vi "NetworkStreamProcess.vi"(0 "WaveformConfiguration":T1, 11 "error in (no error)":errorcluster) -> ()   [LabVIEW 2017]
uses:
  <vilib>/NI/DCAF/Modules/FPGAWaveform/execution/Export.ctl
  StreamState.ctl
  StreamHeader.ctl
  globals.vi
  <vilib>/NI/DCAF/Modules/FPGAWaveform/execution/WaveformAcq runtime.lvclass
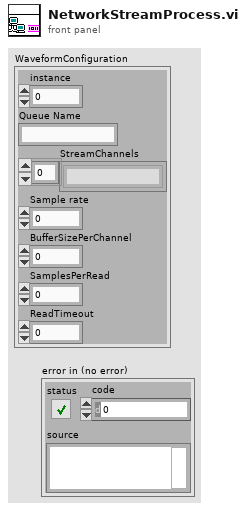
[diagram p1: front panel]
types:
  T1 = typedef "WaveformAcq runtime.lvclass/Export.ctl" = cluster{"instance":i32, "Queue Name":string, "StreamChannels":string[], "Sample rate":i32, "BufferSizePerChannel":i32, "SamplesPerRead":i32, "ReadTimeout":dbl}
  T2 = typedef "StreamHeader.ctl" = cluster{"Channels":string[], "SampleRate":i32}
  T3 = typedef "StreamState.ctl" = enum16{"Idle", "Listening", "Header", "Streaming", "Disconnecting"}
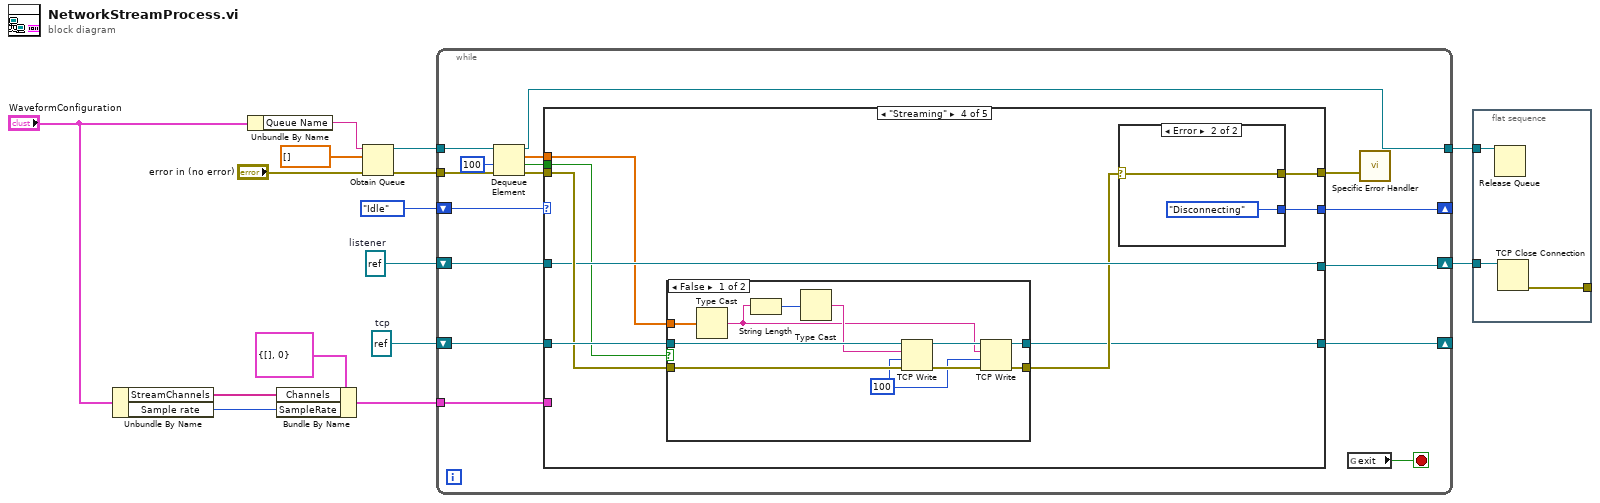
[diagram p0: block diagram]
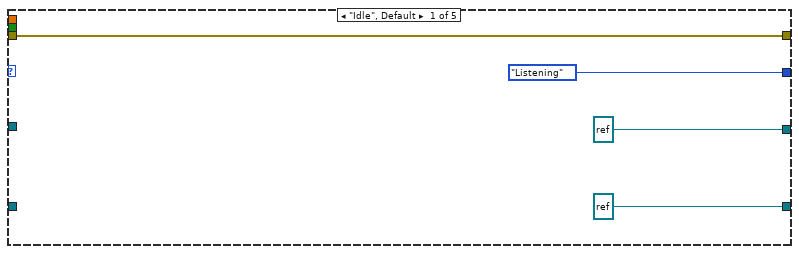
[diagram p2: hidden frame]
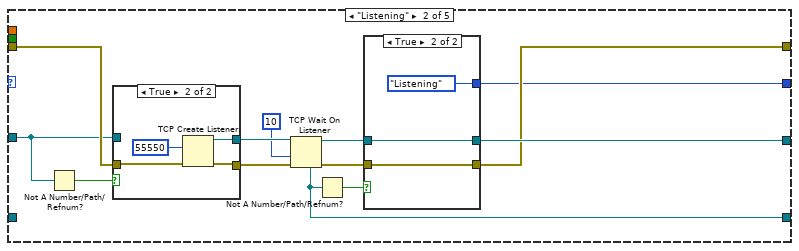
[diagram p3: hidden frame]
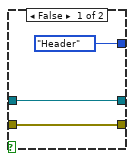
[diagram p4: hidden frame]
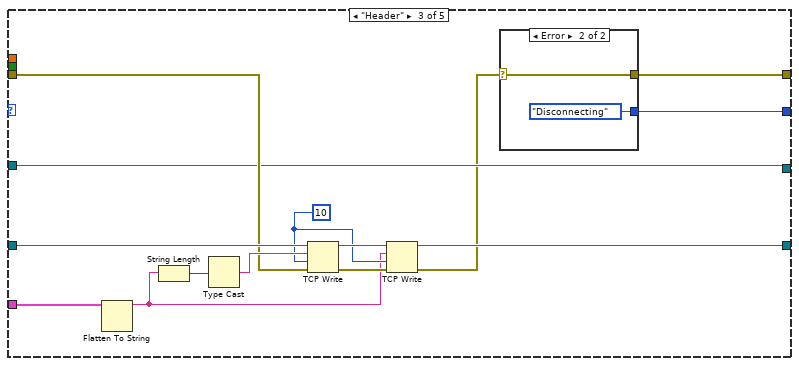
[diagram p6: hidden frame]
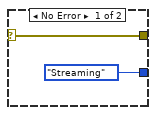
[diagram p7: hidden frame]
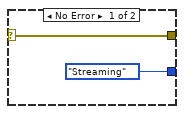
[diagram p8: hidden frame]
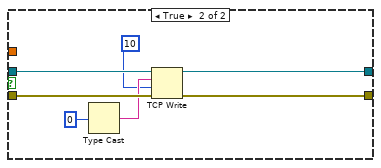
[diagram p9: hidden frame]
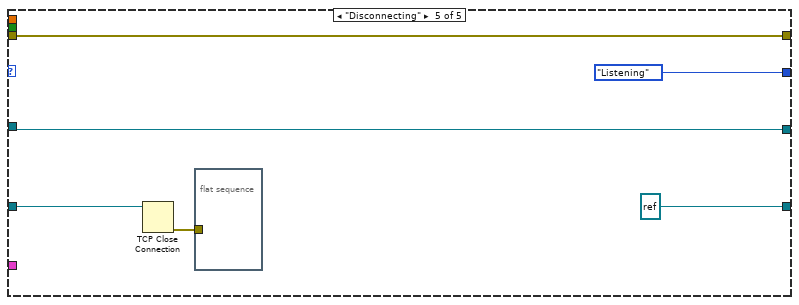
[diagram p10: hidden frame]
diagram:
  w8 = refnum<k5> refnum  # tcp
  w9 = refnum<k5> refnum  # listener
  n1 = Unbundle By Name("WaveformConfiguration") -> ("StreamChannels"=w3:string[], "Sample rate"=w2:i32)
  n2 = Unbundle By Name("WaveformConfiguration") -> ("Queue Name"=w7:string)
  n3 = Bundle By Name(cluster=T2 {"Channels"=[], "SampleRate"=0} ("StreamHeader"), "Channels"=w3, "SampleRate"=w2) -> (w4:T2)
  n4 = Obtain Queue(name (unnamed)=w7, element data type=sgl[] [], error in (no error)="error in (no error)") -> (queue out=w13:refnum<queue>, error out=w14:errorcluster)  [unwired: 2 in, 1 out]
  n5 = while {
    tunnel: w13 -> [w31]
    tunnel: w14 -> [w30]
    tunnel: [w28] -> w15
    shift-right: [w24] -> _
    shift-left: StreamState."Idle" ("StreamState") -> [w26]
    shift-right: [w19] -> w1
    shift-left: w9 -> [w22]
    shift-right: [w18] -> _
    shift-left: w8 -> [w17]
    tunnel: w4 -> [w16]
    stop <- w27 stop-if-true
    n6 = Dequeue Element(queue=w31, timeout in ms (-1)=100, error in (no error)=w30) -> (queue out=w28:refnum<queue>, element=w20:sgl[], timed out?=w21:bool, error out=w25:errorcluster)
    n7 = case shown="\"Streaming\"" w26 {
      tunnel: w25 -> [w32 w47 w71 w86 w111]
      tunnel: [StreamState."Listening" ("StreamState") w36 w67 w85 StreamState."Listening" ("StreamState")] -> w24
      tunnel: [w32 w37 w63 w80 w111] -> w23
      tunnel: w22 -> [_ w46 w65 w84 w110]
      tunnel: w21 -> [_ _ _ w83 _]
      tunnel: w20 -> [_ _ _ w82 _]
      tunnel: [refnum<k5> refnum ("listener ID") w39 w65 w84 w110] -> w19
      tunnel: [refnum<k5> refnum ("listener ID") w38 w66 w79 refnum<k5> refnum ("tcp")] -> w18
      tunnel: w17 -> [_ _ w74 w87 w115]
      tunnel: w16 -> [_ _ w62 _ _]
      frame "Idle", Default {
      }
      frame "Listening" {
        n8 = Not A Number/Path/Refnum?(number/path/refnum=w46) -> (NaN/Path/Refnum?=w48:bool)
        n9 = case shown="True" w48 {
          tunnel: w47 -> [w55 w60]
          tunnel: [w56 w59] -> w45
          tunnel: w46 -> [w56 _]
          tunnel: [w55 w58] -> w44
          frame False {
          }
          frame True {
            n10 = TCP Create Listener(8:w60, 10:u16 55550 ("port")) -> (0:w58:errorcluster, 3:w59:refnum<k5>)  [unwired: 3 in, 1 out]
          }
        }
        n11 = TCP Wait On Listener(8:w44, 9:10 ("timeout ms (wait forever: -1)"), 11:w45) -> (0:w41:errorcluster, 3:w40:refnum<k5>, 4:w38:refnum<k5>)  [unwired: 1 in, 2 out]
        n12 = Not A Number/Path/Refnum?(number/path/refnum=w38) -> (NaN/Path/Refnum?=w42:bool)
        n13 = case shown="True" w42 {
          tunnel: w41 -> [w49 w53]
          tunnel: w40 -> [w50 w54]
          tunnel: [w50 w54] -> w39
          tunnel: [w49 w53] -> w37
          tunnel: [StreamState."Header" ("StreamState") StreamState."Listening" ("StreamState")] -> w36
          frame False {
          }
          frame True {
          }
        }
      }
      frame "Header" {
        w68 = 10 ("timeout ms (25000)")
        n14 = Flatten To String(anything=w62) -> (data string=w61:string)  [unwired: 3 in, 2 out]
        n15 = String Length(string=w61) -> (length=w73:i32)
        n16 = Type Cast(x=w73) -> (*(type *) &x=w72:string)  [unwired: 1 in]
        n17 = TCP Write(connection ID=w74, data in=w72, error in (no error)=w71, 9:w68) -> (connection ID out=w70:refnum<k5>, error out=w69:errorcluster)  [unwired: 1 out]
        n18 = TCP Write(connection ID=w70, data in=w61, error in (no error)=w69, 9:w68) -> (connection ID out=w66:refnum<k5>, error out=w64:errorcluster)  [unwired: 1 out]
        n19 = case shown="Error" w64 {
          selector: w64 -> [w75 w78]
          tunnel: [StreamState."Streaming" ("StreamState") StreamState."Disconnecting" ("StreamState")] -> w67
          tunnel: [w75 w78] -> w63
          frame No Error {
          }
          frame Error {
          }
        }
      }
      frame "Streaming" {
        n20 = case shown="False" w83 {
          tunnel: w87 -> [w102 w109]
          tunnel: w86 -> [w99 w108]
          tunnel: [w95 w107] -> w81
          tunnel: [w94 w106] -> w79
          tunnel: w82 -> [w93 _]
          frame False {
            w96 = 100 ("timeout ms (25000)")
            n21 = Type Cast(x=w93) -> (*(type *) &x=w92:string)  [unwired: 1 in]
            n22 = String Length(string=w92) -> (length=w101:i32)
            n23 = Type Cast(x=w101) -> (*(type *) &x=w100:string)  [unwired: 1 in]
            n24 = TCP Write(connection ID=w102, data in=w100, error in (no error)=w99, 9:w96) -> (connection ID out=w98:refnum<k5>, error out=w97:errorcluster)  [unwired: 1 out]
            n25 = TCP Write(connection ID=w98, data in=w92, error in (no error)=w97, 9:w96) -> (connection ID out=w94:refnum<k5>, error out=w95:errorcluster)  [unwired: 1 out]
          }
          frame True {
            n26 = Type Cast(x=0) -> (*(type *) &x=w104:string)  [unwired: 1 in]
            n27 = TCP Write(connection ID=w109, data in=w104, error in (no error)=w108, 9:10 ("timeout ms (25000)")) -> (connection ID out=w106:refnum<k5>, error out=w107:errorcluster)  [unwired: 1 out]
          }
        }
        n28 = case shown="Error" w81 {
          selector: w81 -> [w88 w91]
          tunnel: [StreamState."Streaming" ("StreamState") StreamState."Disconnecting" ("StreamState")] -> w85
          tunnel: [w88 w91] -> w80
          frame No Error {
          }
          frame Error {
          }
        }
      }
      frame "Disconnecting" {
        n29 = TCP Close Connection(connection ID=w115) -> (error out=w113:errorcluster)  [unwired: 2 in, 1 out]
        n30 = flat-sequence {
          tunnel: w113 -> [_]
          frame #0 {
          }
        }
      }
    }
    n31 = global read "globals.vi" "exit"() -> (w27:bool)
    n32 = call "Specific Error Handler"("Error to Check"=w23) -> ()  [unwired: 11 in, 4 out]
  }
  n33 = flat-sequence {
    tunnel: w15 -> [w118]
    tunnel: w1 -> [w117]
    tunnel: [w116] -> _
    frame #0 {
      n34 = Release Queue(queue=w118) -> ()  [unwired: 2 in, 3 out]
      n35 = TCP Close Connection(connection ID=w117) -> (error out=w116:errorcluster)  [unwired: 2 in, 1 out]
    }
  }
